vi "Configure List Sweep.vi"(5 "Sweep List Data Type (0: Append)":i32(ring) items=["Append", "New List"], 6 "Sweep List Start Index (1)":i32=1, 7 "Source Type (1: Fixed)":i32(ring)=1 items=["Arbitrary", "Fixed", "Sweep", "List"], 8 "error in (no error)":errorcluster, 9 "Sweep List Data":dbl[](array[numeric]), 10 "Channel (1: Channel 1)":i32(ring)=1 items=["Channel 1"=1, "Channel 2"=2], 11 "VISA resource name":refnum<visa-resource-name>) -> (0 "error out":errorcluster, 3 "VISA resource name out":refnum<visa-resource-name>)   [LabVIEW 2012, in "Keysight B2980 Series.lvlib"]
doc: "Configures settings for list sweep.\n\n<b>Note(s):</b>\nThis VI is only applicable for model B2985A and B2987A."
uses:
  Keysight B2980 Series.lvlib
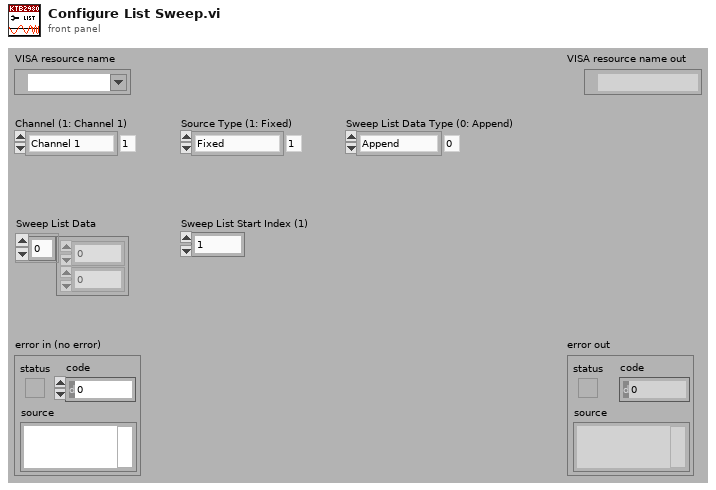
[diagram p1: front panel]
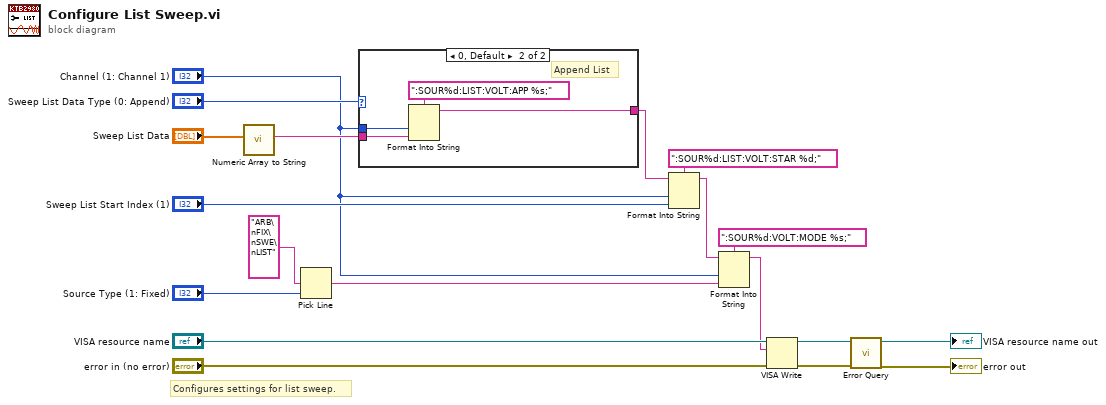
[diagram p0: block diagram]
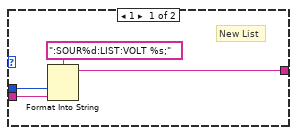
[diagram p2: hidden frame]
diagram:
  # "Configures settings for list sweep."
  n1 = call "Numeric Array to String.vi"("List Data"="Sweep List Data") -> ("Result String"=w7:string)  [unwired: 10 out]
  n2 = Pick Line(multi-line string="ARB\nFIX\nSWE\nLIST", line index="Source Type (1: Fixed)") -> (output string=w14:string)  [unwired: 1 out]
  n3 = case shown="0, Default" "Sweep List Data Type (0: Append)" {
    tunnel: "Channel (1: Channel 1)" -> [w22 w26]
    tunnel: w7 -> [w21 w25]
    tunnel: [w20 w24] -> w6
    frame 1 {
      # "New List"
      n4 = Format Into String(format string=":SOUR%d:LIST:VOLT %s;", w22, w21) -> (resulting string=w20:string)  [unwired: 2 in, 1 out]
    }
    frame 0, Default {
      # "Append List"
      n5 = Format Into String(format string=":SOUR%d:LIST:VOLT:APP %s;", w26, w25) -> (resulting string=w24:string)  [unwired: 2 in, 1 out]
    }
  }
  n6 = Format Into String(format string=":SOUR%d:LIST:VOLT:STAR %d;", initial string=w6, "Channel (1: Channel 1)", "Sweep List Start Index (1)") -> (resulting string=w5:string)  [unwired: 1 in, 1 out]
  n7 = Format Into String(format string=":SOUR%d:VOLT:MODE %s;", initial string=w5, "Channel (1: Channel 1)", w14) -> (resulting string=w4:string)  [unwired: 1 in, 1 out]
  n8 = VISA Write(VISA resource name="VISA resource name", write buffer=w4, error in (no error)="error in (no error)") -> (VISA resource name out=w2:refnum<visa-resource-name>, error out=w1:errorcluster)  [unwired: 1 out]
  n9 = call "Error Query.vi"("error in (no error)"=w1, "VISA resource name"=w2) -> ("error out"=→"error out":errorcluster, "VISA resource name out"=→"VISA resource name out":refnum<visa-resource-name>)  [unwired: 8 out]
